vi "Close.vi"(0 "PM NI568X in":refnum<class "Power Meter.lvclass">, 11 "error in (no error)":errorcluster) -> (4 "PM NI568X out":refnum<class "Power Meter.lvclass">, 15 "error out":errorcluster)   [LabVIEW 2023, in "NI-568x RF Power Meter.lvlib" / "Power Meter.lvclass"]
uses:
  Power Meter.lvclass
  Power Meter.lvclass/Power Meter.ctl
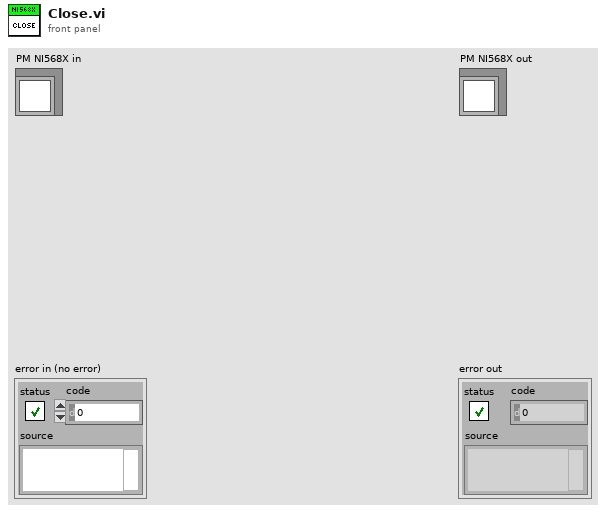
[diagram p1: front panel]
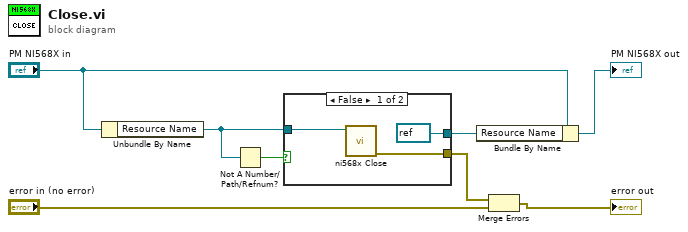
[diagram p0: block diagram]
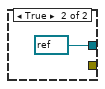
[diagram p2: hidden frame]
diagram:
  n1 = Unbundle By Name("PM NI568X in") -> ("Resource Name"=w4:refnum<k15>)
  n2 = Not A Number/Path/Refnum?(number/path/refnum=w4) -> (NaN/Path/Refnum?=w8:bool)
  n3 = case shown="False" w8 {
    tunnel: w4 -> [w11 _]
    tunnel: [refnum<k15> refnum ("Resource Name") refnum<k15> refnum ("Resource Name")] -> w2
    tunnel: [w9 _] -> w7
    frame False {
      n4 = call <instrlib>:"ni568x Close.vi"("instrument handle"=w11) -> ("error out"=w9:errorcluster)  [unwired: 10 in]
    }
    frame True {
    }
  }
  n5 = Bundle By Name(cluster="PM NI568X in", "Resource Name"=w2) -> (→"PM NI568X out":refnum<class "Power Meter.lvclass">)
  n6 = Merge Errors(w7, "error in (no error)") -> (→"error out":errorcluster)
